vi "_Set Scan Type.vi"(0 "ScanType Offset":u16) -> ()   [LabVIEW 2012]
uses:
  Type/_FPGA DC Lines.ctl
  <vilib>/rvi/DataTransferAndStorage/Container/Common/niFpgaContainerGetUniqueNameForEmu.vi
  <vilib>/rvi/Memory/Memory_Emulation/niFpgaMemoryEmulationCacheClearOnFirstRun.vi
  <vilib>/rvi/Memory/Memory_Emulation/nirvimemoryEmulationManagerCache_MakeExclusive.vi
  <vilib>/rvi/Memory/Memory_Emulation/niFpgaMemoryEmulationValidateCache.vi
  <vilib>/rvi/Memory/Memory_Emulation/nirvimemoryEmulationManagerCache_ReleaseExclusive.vi
  <vilib>/rvi/Memory/Memory_Emulation/nirvimemoryEmulationManagerCache_InsertValue.vi
  <vilib>/Utility/error.llb/Clear Errors.vi
  <vilib>/rvi/Memory/Memory_Emulation/nirvimemoryEmulationManagerCache_GetValue.vi
  <vilib>/rvi/DataTransferAndStorage/Container/XNode/niFpgaContainer.xnode
  <vilib>/rvi/Memory/Memory_Emulation/nirvimemoryEmulation.vi
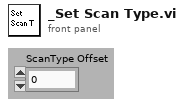
[diagram p1: front panel]
types:
  T1 = typedef "_FPGA DC Lines.ctl" = enum16{"Q1 POL", "Q3 POL", "Q1 DC EN", "Q3 DC EN", "COR POL", "CUR POL", "S1 POL", "S2 POL", "CEM POL"}
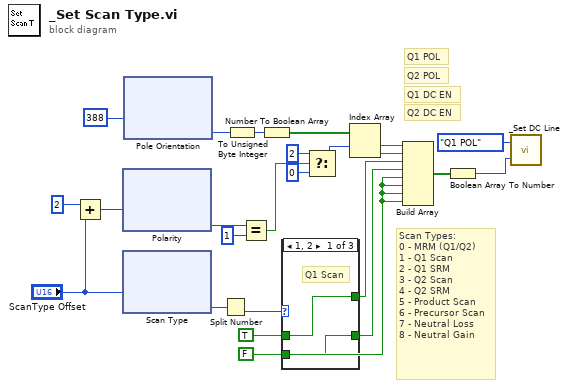
[diagram p0: block diagram]
diagram:
  w19 = FALSE
  # "Q2 DC EN"
  # "Q1 DC EN"
  # "Q2 POL"
  # "Q1 POL"
  # "Scan Types:\n0 - MRM (Q1/Q2)\n1 - Q1 Scan\n2 - Q1 SRM\n3 - Q2 Scan\n4 - Q2 SRM\n5 - Product Scan\n6 - Precursor Scan\n7 - Neutral Loss\n8 - Neutral Gain"
  n1 = Add(x=u16 2, y="ScanType Offset") -> (x+y=w12:u16)
  n2 = xnode "Polarity"("Address"=w12) -> ("Data"=w8:u32)  [unwired: 1 in, 1 out]
  n3 = xnode "Scan Type"("Address"="ScanType Offset") -> ("Data"=w17:u32)  [unwired: 1 in, 1 out]
  n4 = xnode "Pole Orientation"("Address"=u16 388) -> ("Data"=w14:u32)  [unwired: 1 in, 1 out]
  n5 = Split Number(x=w17) -> (lo(x)=w16:u16)  [unwired: 1 out]
  n6 = To Unsigned Byte Integer(number=w14) -> (unsigned 8bit integer=w13:u8)
  n7 = Equal?(x=w8, y=u8 1) -> (x = y?=w1:bool)
  n8 = Number To Boolean Array(number=w13) -> (Boolean array=w7:bool[])
  n9 = case shown="1, 2" w16 {
    tunnel: TRUE -> [w26 w28 w29]
    tunnel: w19 -> [w25 w27 _]
    tunnel: [w26 w27 w29] -> w22
    tunnel: [w25 w28 w29] -> w21
    frame 1, 2 {
      # "Q1 Scan"
    }
    frame 3, 4 {
      # "Q2 Scan"
    }
    frame 0, Default {
      # "MS/MS"
    }
  }
  n10 = Select(t=u8 2 ("y"), s=w1, f=u8 0 ("y")) -> (s? t:f=w2:u8)
  n11 = Index Array(array=w7, index #1=w2) -> (element #1=w6:bool, element #2=w5:bool)  [unwired: 1 in]
  n12 = Build Array(w6, w5, w22, w21, w19, w19, w19, w19) -> (w20:bool[])
  n13 = Boolean Array To Number(Boolean array=w20) -> (number=w18:u8)
  n14 = call "_Set DC Line.vi"("States"=w18, "DC Line"=_FPGA_DC_Lines."Q1 POL") -> ()  [unwired: 2 out]
